vi "Driver - DTACQ - Send Asynchronous Message.vi"(8 "error in":errorcluster, 10 "Message to Send":string, 11 "DTACQ Connection Data In":T1={"Description"="", "Address"="", "Port"=0, "timeout (ms)"=5000, "Termination Character"="\n", "TCP Connection Reference"=refnum, "Open Connection"=FALSE}) -> (0 "error out":errorcluster, 3 "DTACQ Connection Data Out":T1={"Description"="", "Address"="", "Port"=0, "timeout (ms)"=5000, "Termination Character"="\n", "TCP Connection Reference"=refnum, "Open Connection"=FALSE})   [LabVIEW 2017, in "Communications Library.lvlib"]
doc: "Writes a string to a DTACQ device using TCP. Does not wait for a response message.\n\nOpens the TCP connection, if it is not already open."
uses:
  Communications Library.lvlib
  Typedefs/DTACQ Connection Data--Cluster.ctl
  Debug - Lower Level - Logging Tool.vi
  Error 5102 - DTACQ unit replied with an error--const.vi
  <vilib>/Utility/error.llb/Error Cluster From Error Code.vi
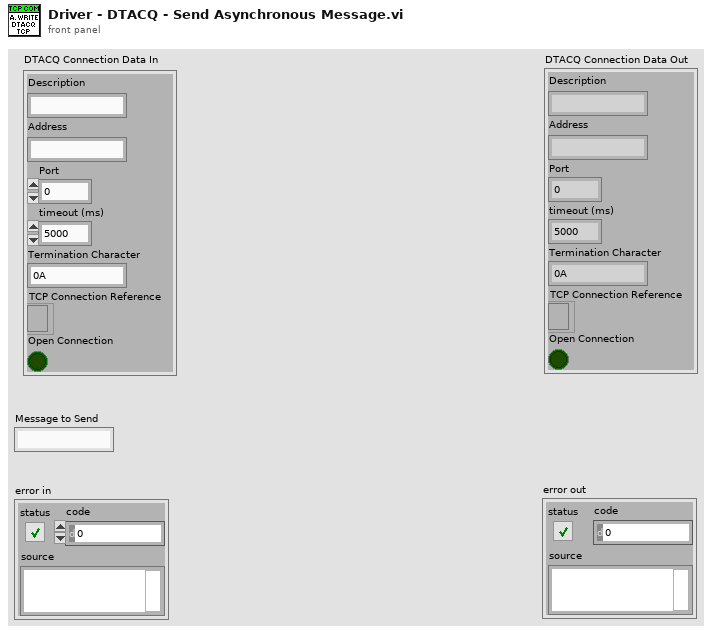
[diagram p1: front panel]
types:
  T1 = typedef "Communications Library.lvlib/DTACQ Connection Data--Cluster.ctl" = cluster{"Description":string, "Address":string, "Port":u16, "timeout (ms)":i32, "Termination Character":string, "TCP Connection Reference":refnum<k5>, "Open Connection":bool}
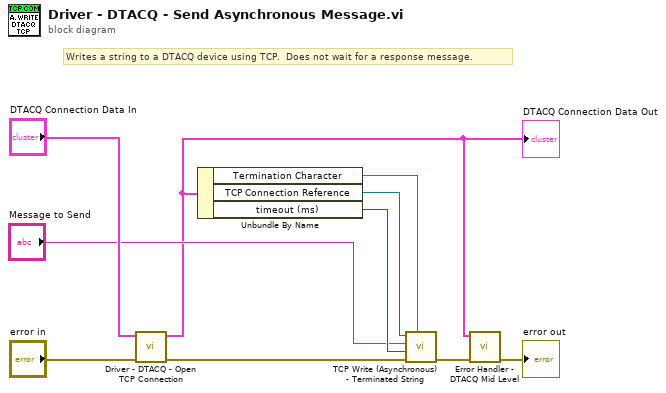
[diagram p0: block diagram]
diagram:
  # "Writes a string to a DTACQ device using TCP.  Does not wait for a response message."
  n1 = call "Driver - DTACQ - Open TCP Connection.vi"("error in"="error in", "DTACQ Connection Data In"="DTACQ Connection Data In") -> ("error out"=w6:errorcluster, "DTACQ Connection Data Out"=w1:T1)  [unwired: 8 in]
  "DTACQ Connection Data Out" <- w1
  n2 = Unbundle By Name(w1) -> ("Termination Character"=w10:string, "TCP Connection Reference"=w9:refnum<k5>, "timeout (ms)"=w8:i32)
  n3 = call "TCP Write (Asynchronous) - Terminated String.vi"("Termination Character"=w10, "error in"=w6, "Timeout ms (default 50ms)"=w8, "Message to Send"="Message to Send", "TCP Network Connection in"=w9) -> ("error out"=w3:errorcluster)  [unwired: 5 in, 1 out]
  n4 = call "Error Handler - DTACQ Mid Level.vi"("error in"=w3, "DTACQ Connection Data In"=w1) -> ("error out"=→"error out":errorcluster)  [unwired: 7 in, 2 out]
